vi "Save_single.vi"(3 "Saved Vis paths in":path[](array[path]), 4 "Top level VI Name":path, 5 "VI to save":path) -> (0 "Saved Vis paths Out":path[](array[path]), 1 "Execution:State":T1(ring), 2 "Error IO":errorcluster)   [LabVIEW 2010]
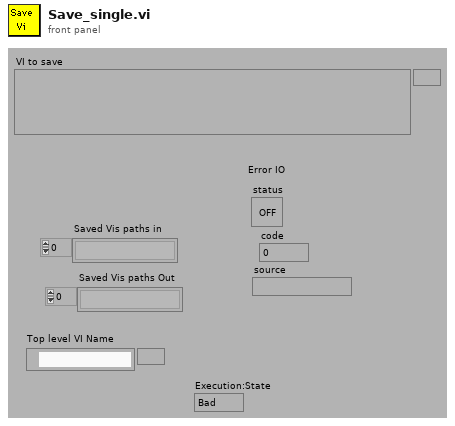
[diagram p1: front panel]
types:
  T1 = enum32{"Bad", "Idle", "Run top level", "Running"}
  T2 = enum32{"invalid VI type", "Standard VI", "Control VI", "Global VI", "Polymorphic VI", "Configuration VI", "SubSystem", "Facade VI", "Method VI", "Statechart Diagram VI"}
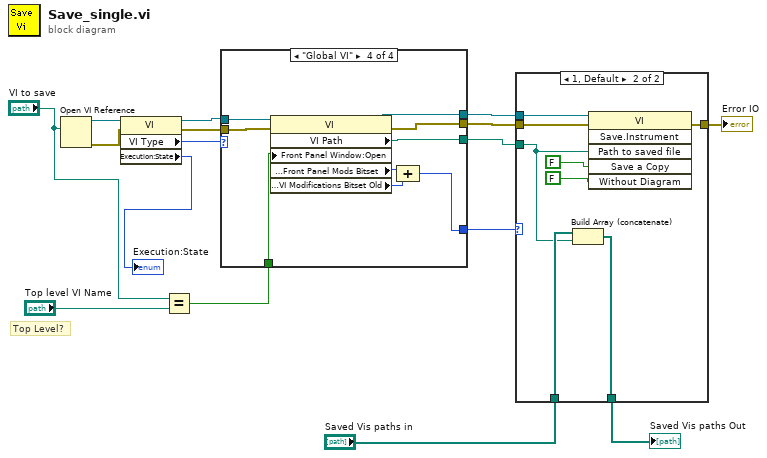
[diagram p0: block diagram]
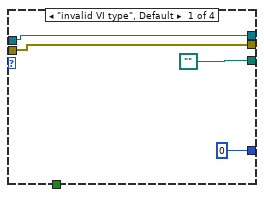
[diagram p2: hidden frame]
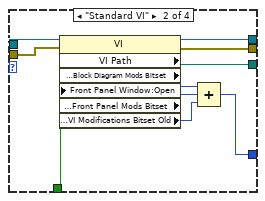
[diagram p3: hidden frame]
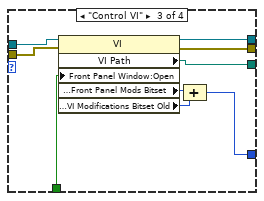
[diagram p4: hidden frame]
diagram:
  # "Top Level?"
  n1 = Open VI Reference(vi path="VI to save") -> (vi reference=w5:refnum<vi>, error out=w4:errorcluster)  [unwired: 5 in]
  n2 = property class="VI"(reference=w5, error in=w4) -> (reference out=w11:refnum<vi>, error out=w10:errorcluster, "VI Type"=w12:T2, "Execution:State"=→"Execution:State":T1)
  n3 = Equal?(x="VI to save", y="Top level VI Name") -> (x = y?=w3:bool)
  n4 = case shown="\"Global VI\"" w12 {
    tunnel: [path "" ("Path") w30 w31 w40] -> w6
    tunnel: [w18 w29 w39 w48] -> w15
    tunnel: [w19 w28 w38 w47] -> w14
    tunnel: w11 -> [w18 w27 w37 w46]
    tunnel: [u32 0 w25 w33 w42] -> w13
    tunnel: w10 -> [w19 w26 w36 w45]
    tunnel: w3 -> [_ w24 w32 w41]
    frame "invalid VI type", Default {
    }
    frame "Standard VI" {
      n5 = property class="VI"(reference=w27, error in=w26, "Front Panel Window:Open"=w24) -> (reference out=w29:refnum<vi>, error out=w28:errorcluster, "VI Path"=w30:path, "Modifications:Block Diagram Mods Bitset"=w23:u32, "Modifications:Front Panel Mods Bitset"=w22:u32, "Modifications:VI Modifications Bitset Old"=w21:u32)
      n6 = Compound Arithmetic op=ADD(w23, w22, w21) -> (w25:u32)
    }
    frame "Control VI" {
      n7 = property class="VI"(reference=w37, error in=w36, "Front Panel Window:Open"=w32) -> (reference out=w39:refnum<vi>, error out=w38:errorcluster, "VI Path"=w31:path, "Modifications:Front Panel Mods Bitset"=w35:u32, "Modifications:VI Modifications Bitset Old"=w34:u32)
      n8 = Compound Arithmetic op=ADD(w35, w34) -> (w33:u32)
    }
    frame "Global VI" {
      n9 = property class="VI"(reference=w46, error in=w45, "Front Panel Window:Open"=w41) -> (reference out=w48:refnum<vi>, error out=w47:errorcluster, "VI Path"=w40:path, "Modifications:Front Panel Mods Bitset"=w44:u32, "Modifications:VI Modifications Bitset Old"=w43:u32)
      n10 = Compound Arithmetic op=ADD(w44, w43) -> (w42:u32)
    }
  }
  n11 = case shown="1, Default" w13 {
    tunnel: w6 -> [_ w51]
    tunnel: w15 -> [_ w56]
    tunnel: w14 -> [w50 w55]
    tunnel: [w50 w54] -> w7
    tunnel: [w49 w52] -> w9
    tunnel: "Saved Vis paths in" -> [w49 w53]
    frame 0 {
    }
    frame 1, Default {
      n12 = Build Array (concatenate)(w53, w51) -> (w52:path[])
      n13 = invoke class="VI" method="Save.Instrument"(reference=w56, error in=w55, "Path to saved file"=w51, "Save a Copy"=FALSE, "Without Diagram"=FALSE) -> (error out=w54:errorcluster)  [unwired: 1 in, 5 out]
    }
  }
  "Error IO" <- w7
  "Saved Vis paths Out" <- w9
